vi "EMV Sample History.vi"(8 "error in (no error)":errorcluster, 11 "T6 Temp":dbl) -> (0 "error out":errorcluster, 3 "T6 History":dbl[](array[numeric]))   [LabVIEW 2016]
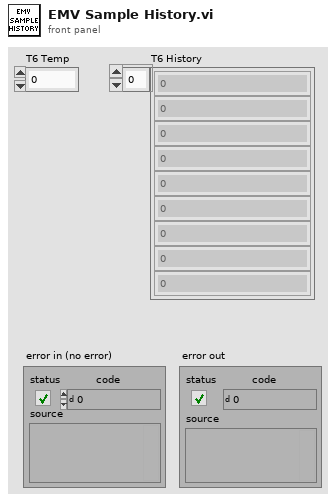
[diagram p1: front panel]
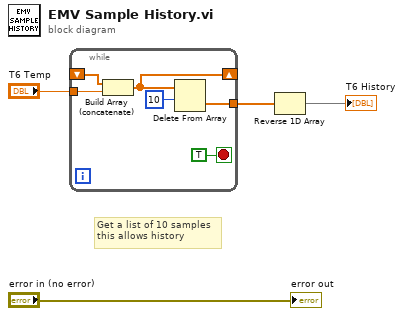
[diagram p0: block diagram]
diagram:
  # "Get a list of 10 samples \nthis allows history"
  n1 = while {
    shift-right: [w8] -> _
    shift-left: _ -> [w10]
    tunnel: "T6 Temp" -> [w6]
    tunnel: [w5] -> w2
    stop <- TRUE stop-if-true
    n2 = Build Array (concatenate)(w10, w6) -> (w8:dbl[])
    n3 = Delete From Array(array=w8, length=10) -> (deleted portion=w5:dbl[])  [unwired: 1 in, 1 out]
  }
  n4 = Reverse 1D Array(array=w2) -> (reversed array=→"T6 History":dbl[])
  "error out" <- "error in (no error)"
